vi "controle energie.vi"(7 "Date Fin":timestamp format="%<%.0X %x>T", 8 "Error in (no error)":errorcluster, 9 "Date Debut":timestamp format="%<%.0X %x>T", 10 "ID compresseur":dbl, 11 "Connection In":refnum<k7>) -> (0 "Error out":errorcluster, 1 "Temp":dbl, 2 "Emergie":dbl, 3 "Connection Out":refnum<k7>)   [LabVIEW 2019]
panel:
  out "concatenated string":string
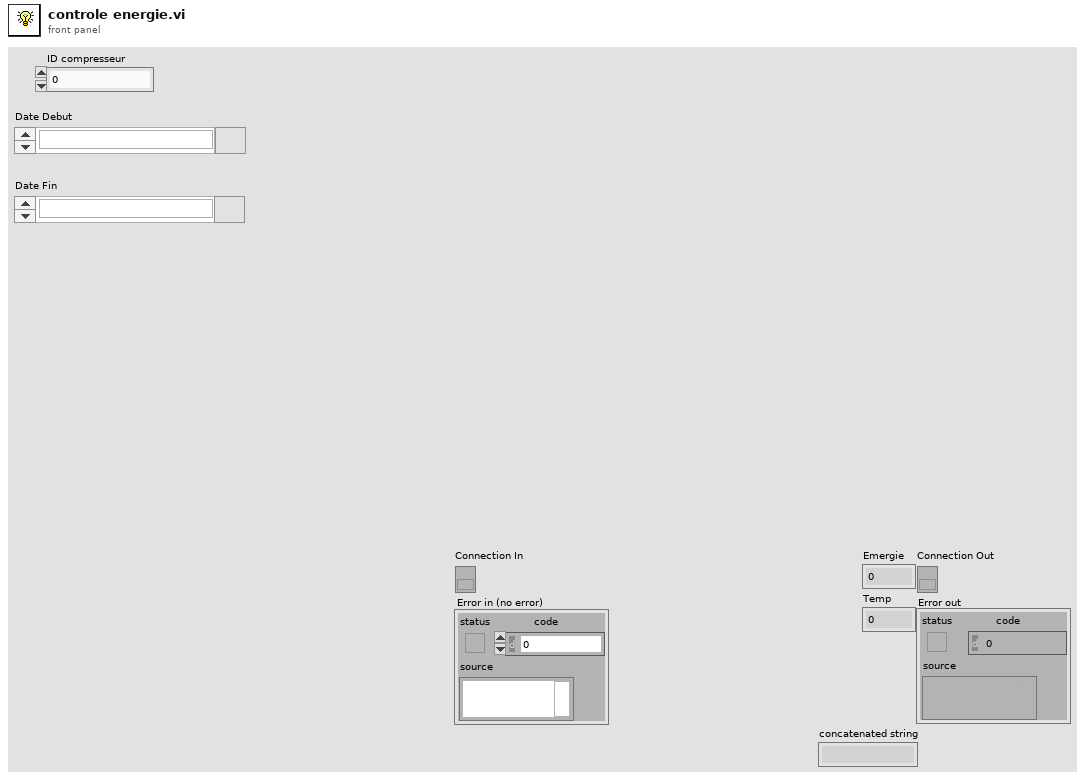
[diagram p1: front panel]
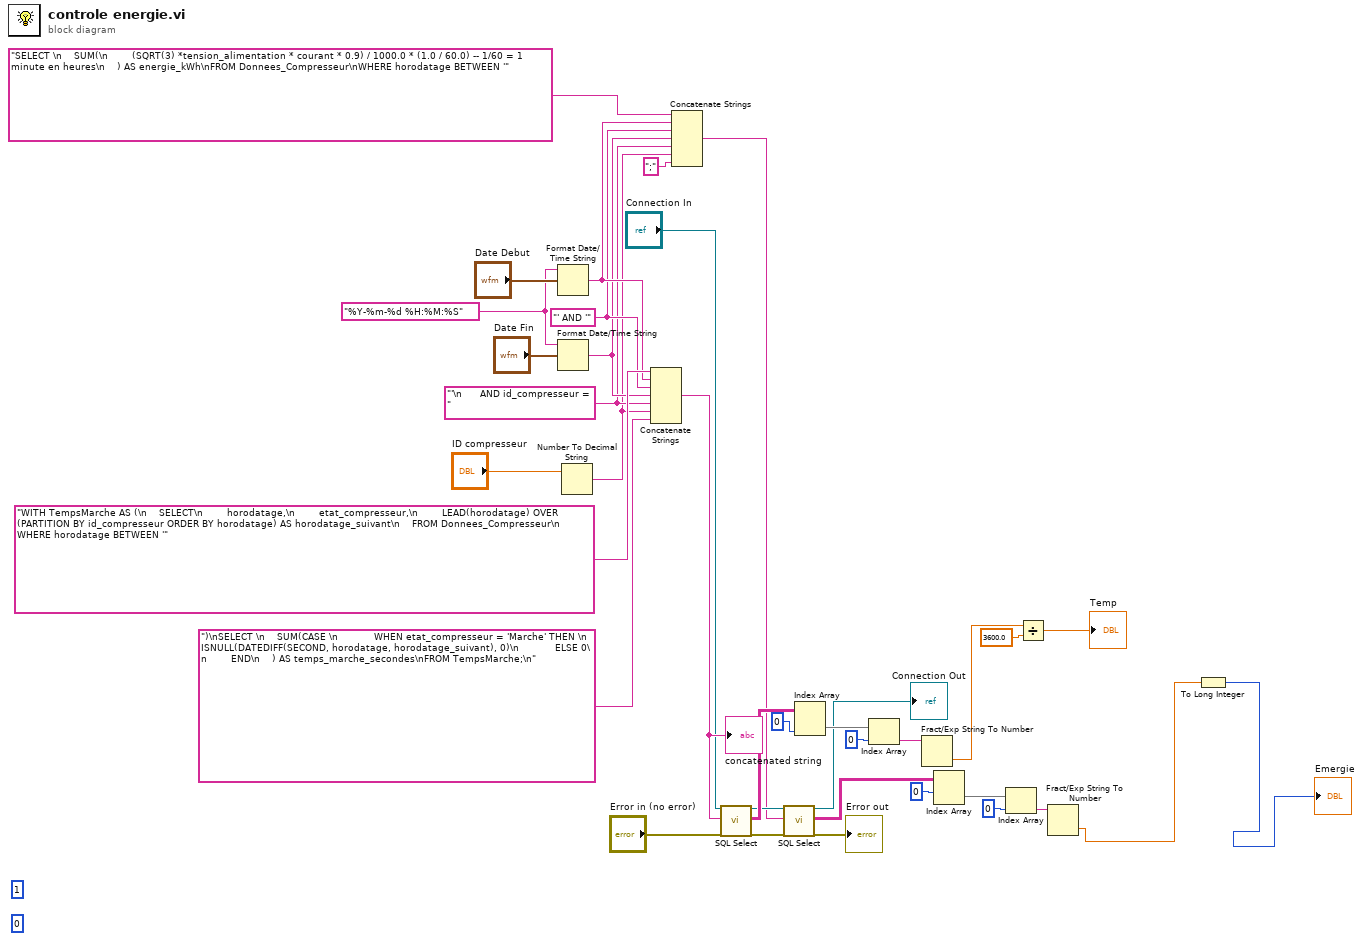
[diagram p0: block diagram]
diagram:
  (unwired) 0 ("index")
  (unwired) 1 ("index (row)")
  w12 = "'\n      AND id_compresseur = " ("string")
  w14 = "' AND '" ("string")
  w28 = "%Y-%m-%d %H:%M:%S" ("time format string (%c)")
  n1 = Format Date/Time String(time format string (%c)=w28, seconds (now)="Date Debut") -> (date/time string=w15:string)  [unwired: 1 in]
  n2 = Format Date/Time String(time format string (%c)=w28, seconds (now)="Date Fin") -> (date/time string=w13:string)  [unwired: 1 in]
  n3 = Number To Decimal String(number="ID compresseur") -> (decimal integer string=w11:string)  [unwired: 1 in]
  n4 = Concatenate Strings("WITH TempsMarche AS (\n    SELECT\n        horodatage,\n        etat_compresseur,\n        LEAD(horodatage) OVER (PARTITION BY id_compresseur ORDER BY horodatage) AS horodatage_suivant\n    FROM Donnees_Compresseur\n    WHERE horodatage BETWEEN '" ("SQL Query"), w15, w14, w13, w12, w11, ")\nSELECT \n    SUM(CASE \n            WHEN etat_compresseur = 'Marche' THEN \n                ISNULL(DATEDIFF(SECOND, horodatage, horodatage_suivant), 0)\n            ELSE 0\n        END\n    ) AS temps_marche_secondes\nFROM TempsMarche;\n" ("string")) -> (w24:string)
  "concatenated string" <- w24
  n5 = Concatenate Strings("SELECT \n    SUM(\n        (SQRT(3) *tension_alimentation * courant * 0.9) / 1000.0 * (1.0 / 60.0) -- 1/60 = 1 minute en heures\n    ) AS energie_kWh\nFROM Donnees_Compresseur\nWHERE horodatage BETWEEN '", w15, w14, w13, w12, w11, ";" ("string")) -> (w16:string)
  n6 = call <vilib>:"SQL Select.vi"("Connection In"="Connection In", "SQL Query"=w24, "Error in (no error)"="Error in (no error)") -> ("Connection Out"=w21:refnum<k7>, "Data"=w31:string[][], "Error out"=w19:errorcluster)  [unwired: 14 in]
  n7 = call <vilib>:"SQL Select.vi"("Connection In"=w21, "SQL Query"=w16, "Error in (no error)"=w19) -> ("Connection Out"=→"Connection Out":refnum<k7>, "Data"=w7:string[][], "Error out"=→"Error out":errorcluster)  [unwired: 14 in]
  n8 = Index Array(array=w31, index (col)=0 ("disabled index (col)")) -> (element=w35:string[])  [unwired: 1 in]
  n9 = Index Array(array=w35, index=0) -> (element=w33:string)
  n10 = Fract/Exp String To Number(string=w33) -> (number=w3:dbl)  [unwired: 3 in, 1 out]
  n11 = Index Array(array=w7, index (row)=0) -> (element=w5:string[])  [unwired: 1 in]
  n12 = Index Array(array=w5, index=0) -> (element=w6:string)
  n13 = Divide(x=w3, y=3600.0) -> (x/y=→"Temp":dbl)
  n14 = Fract/Exp String To Number(string=w6) -> (number=w4:dbl)  [unwired: 3 in, 1 out]
  n15 = To Long Integer(number=w4) -> (32bit integer=→"Emergie":i32)
